vi "GetPositionCategory.vi"(8 "error in (no error)":errorcluster, 11 "RingItem in":refnum<class "RingItem.lvclass">) -> (0 "error out":errorcluster, 2 "position":T1, 3 "RingItem out":refnum<class "RingItem.lvclass">)   [LabVIEW 2009, in "NavScreen.lvlib" / "RingItem.lvclass"]
uses:
  RingItem.lvclass
  PositionCategory.ctl
  NavScreen.lvlib
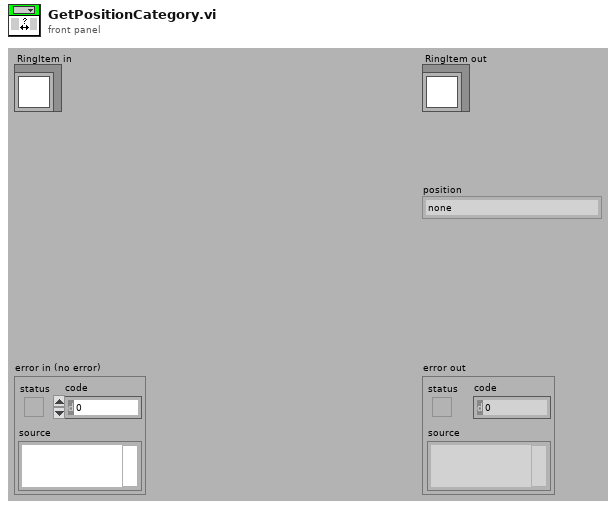
[diagram p1: front panel]
types:
  T1 = typedef "NavScreen.lvlib/PositionCategory.ctl" = enum16{"none", "column 1", "column 2", "ring"}
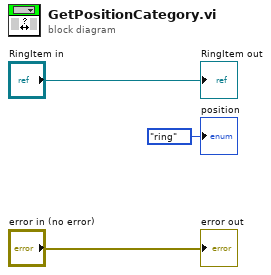
[diagram p0: block diagram]
diagram:
  "error out" <- "error in (no error)"
  "position" <- PositionCategory."ring" ("position")
  "RingItem out" <- "RingItem in"
